vi "Init_Fuente(SubVI).vi"(11 "VISA Refnum in":refnum<visa-resource-name>="GPIB0::5::INSTR") -> (0 "error out":errorcluster, 3 "VISA Refnum out":refnum<visa-resource-name>)   [LabVIEW 2015]
uses:
  <instrlib>/Agilent E364X Series/Agilent E364X Series.lvlib
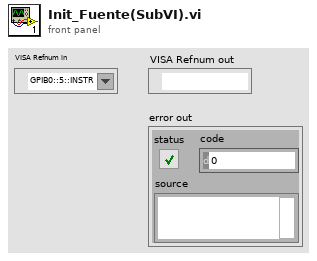
[diagram p1: front panel]
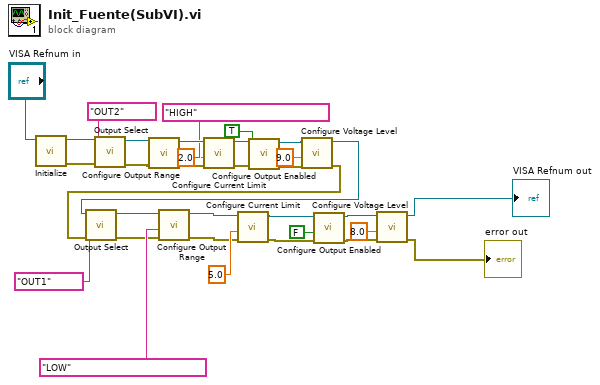
[diagram p0: block diagram]
diagram:
  n1 = call <instrlib>:"Initialize.vi"("VISA resource name"="VISA Refnum in") -> ("error out"=w14:errorcluster, "VISA resource name out"=w15:refnum<visa-resource-name>)  [unwired: 9 in]
  n2 = call <instrlib>:"Output Select.vi"("error in (no error)"=w14, "Instrument Select (Output 1)"="OUT2", "VISA resource name"=w15) -> ("error out"=w12:errorcluster, "VISA resource name out"=w13:refnum<visa-resource-name>)  [unwired: 7 in]
  n3 = call <instrlib>:"Configure Output Range.vi"("error in (no error)"=w12, "Range (High Voltage / Low Current)"="HIGH", "VISA resource name"=w13) -> ("error out"=w10:errorcluster, "VISA resource name out"=w11:refnum<visa-resource-name>)  [unwired: 7 in]
  n4 = call <instrlib>:"Configure Current Limit.vi"("error in (no error)"=w10, "Current Limit (0.0 Amps)"=2.0, "VISA resource name"=w11) -> ("error out"=w8:errorcluster, "VISA resource name out"=w9:refnum<visa-resource-name>)  [unwired: 7 in]
  n5 = call <instrlib>:"Configure Output Enabled.vi"("error in (no error)"=w8, "Output Enabled (F: Off)"=TRUE, "VISA resource name"=w9) -> ("error out"=w6:errorcluster, "VISA resource name out"=w7:refnum<visa-resource-name>)  [unwired: 7 in]
  n6 = call <instrlib>:"Configure Voltage Level.vi"("error in (no error)"=w6, "Level (0.0 Volts)"=9.0, "VISA resource name"=w7) -> ("error out"=w17:errorcluster, "VISA resource name out"=w16:refnum<visa-resource-name>)  [unwired: 7 in]
  n7 = call <instrlib>:"Output Select.vi"("error in (no error)"=w17, "Instrument Select (Output 1)"="OUT1", "VISA resource name"=w16) -> ("error out"=w20:errorcluster, "VISA resource name out"=w19:refnum<visa-resource-name>)  [unwired: 7 in]
  n8 = call <instrlib>:"Configure Output Range.vi"("error in (no error)"=w20, "Range (High Voltage / Low Current)"="LOW", "VISA resource name"=w19) -> ("error out"=w24:errorcluster, "VISA resource name out"=w25:refnum<visa-resource-name>)  [unwired: 7 in]
  n9 = call <instrlib>:"Configure Current Limit.vi"("error in (no error)"=w24, "Current Limit (0.0 Amps)"=5.0, "VISA resource name"=w25) -> ("error out"=w27:errorcluster, "VISA resource name out"=w26:refnum<visa-resource-name>)  [unwired: 7 in]
  n10 = call <instrlib>:"Configure Output Enabled.vi"("error in (no error)"=w27, "Output Enabled (F: Off)"=FALSE, "VISA resource name"=w26) -> ("error out"=w30:errorcluster, "VISA resource name out"=w29:refnum<visa-resource-name>)  [unwired: 7 in]
  n11 = call <instrlib>:"Configure Voltage Level.vi"("error in (no error)"=w30, "Level (0.0 Volts)"=8.0, "VISA resource name"=w29) -> ("error out"=→"error out":errorcluster, "VISA resource name out"=→"VISA Refnum out":refnum<visa-resource-name>)  [unwired: 7 in]
